vi "Read Register Info.vi"(8 "error in (no error)":errorcluster, 11 "CS++PVProxy in":refnum<class "CS++PVProxy.lvclass">) -> (0 "error out":errorcluster, 2 "Register Info":T1(array[cluster]), 3 "CS++PVProxy out":refnum<class "CS++PVProxy.lvclass">)   [LabVIEW 2014, in "CS++PVProxy.lvlib" / "CS++PVProxy.lvclass"]
uses:
  CS++PVProxy.lvclass
  <vilib>/ActorFramework/Message Enqueuer/Message Enqueuer.lvclass
  CS++PVMonitor Messages/CS++PVUpdate Msg/CS++PVUpdate Msg.lvclass
  CS++PVProxy.lvclass/CS++PVProxy.ctl
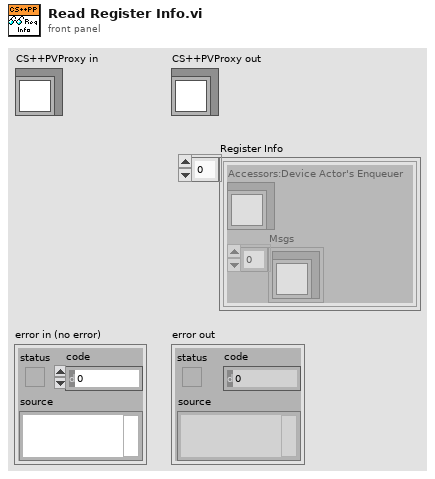
[diagram p1: front panel]
types:
  T1 = cluster{"Accessors:Device Actor's Enqueuer":refnum<class "Message Enqueuer.lvclass">, "Msgs":refnum<class "CS++PVUpdate Msg.lvclass">[]}[]
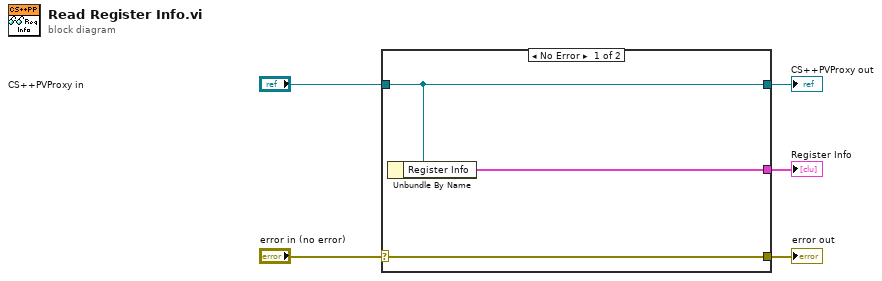
[diagram p0: block diagram]
diagram:
  n1 = case shown="No Error" "error in (no error)" {
    selector: "error in (no error)" -> [w8 w9]
    tunnel: [w8 w9] -> w4
    tunnel: [w7 w10] -> w2
    tunnel: "CS++PVProxy in" -> [w7 w10]
    tunnel: [w6 _] -> w1
    frame No Error {
      n2 = Unbundle By Name(w7) -> ("Register Info"=w6:T1)
    }
    frame Error {
    }
  }
  "error out" <- w4
  "CS++PVProxy out" <- w2
  "Register Info" <- w1
